vi "sync.vi"(1 "LabVIEW Web Service Request":refnum<class "Web Request.lvclass">) -> (4 "status":bool, 6 "source":string, 8 "code":i32)   [LabVIEW 2019]
uses:
  <vilib>/wsapi/Web Request.lvclass
  <vilib>/Utility/file.llb/Read Delimited Spreadsheet (string).vi
  <vilib>/Utility/file.llb/Write Delimited Spreadsheet (string).vi
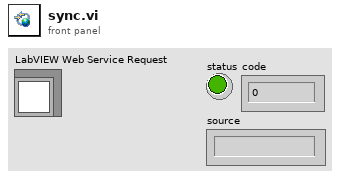
[diagram p1: front panel]
types:
  T1 = cluster{"Local File Path":string, "Client File Name":string, "Content Type":string, "Size":u32}[]
  T2 = cluster{"Local File Path":string, "Client File Name":string, "Content Type":string, "Size":u32}
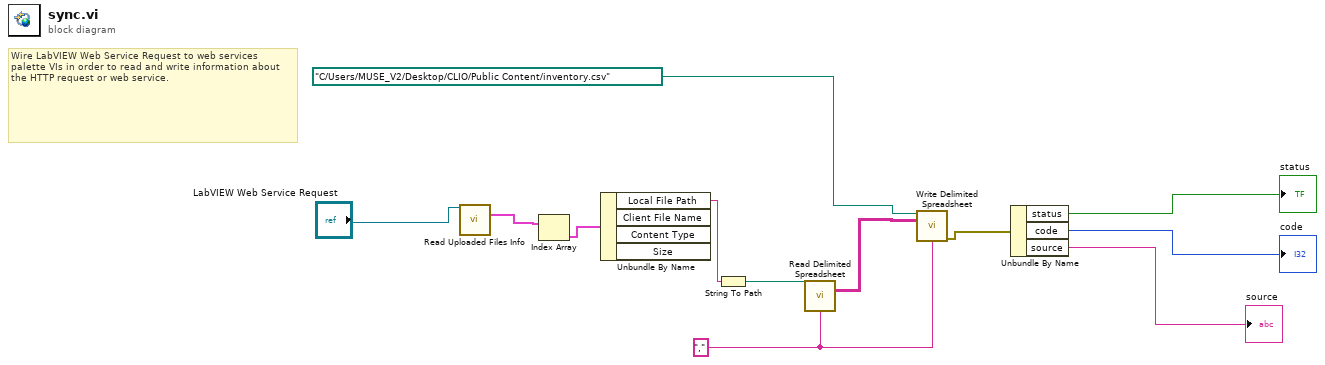
[diagram p0: block diagram]
diagram:
  w5 = ","
  # "Wire LabVIEW Web Service Request to web services palette VIs in order to read and write information about the HTTP request or web service."
  n1 = call <vilib>:"Read Uploaded Files Info.vi"("LabVIEW Web Service Request"="LabVIEW Web Service Request") -> ("UploadedFilesList"=w11:T1)  [unwired: 12 in, 2 out]
  n2 = Index Array(array=w11) -> (element=w10:T2)  [unwired: 1 in]
  n3 = Unbundle By Name(w10) -> ("Local File Path"=w9:string)  [unwired: 3 out]
  n4 = String To Path(string=w9) -> (path=w8:path)
  n5 = call-poly <vilib>:"Read Delimited Spreadsheet.vi"("file path (dialog if empty)"=w8, "delimiter (\\t)"=w5) -> ("all rows"=w6:string[][])  [unwired: 8 in, 5 out]
  n6 = call-poly <vilib>:"Write Delimited Spreadsheet.vi"("file path (dialog if empty)"=path "C:/Users/MUSE_V2/Desktop/CLIO/Public Content/inventory.csv", "2D data"=w6, "delimiter (\\t)"=w5) -> ("error out"=w4:errorcluster)  [unwired: 11 in, 1 out]
  n7 = Unbundle By Name(w4) -> ("status"=→"status":bool, "code"=→"code":i32, "source"=→"source":string)
